vi "minimumSearch.vi"(7 "reset":bool, 11 "input":i16) -> (3 "minimum":i16)   [LabVIEW 2016]
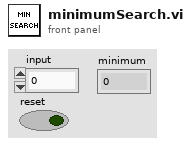
[diagram p1: front panel]
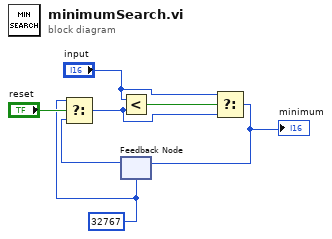
[diagram p0: block diagram]
diagram:
  w1 = i16 32767
  n1 = feedback #1(w1) -> (w5:i16)
  n2 = Select(t=w1, s="reset", f=w5) -> (s? t:f=w3:i16)
  n3 = Less?(x="input", y=w3) -> (x < y?=w7:bool)
  n4 = Select(t="input", s=w7, f=w3) -> (s? t:f=w4:i16)
  "minimum" <- w4
  n5 = feedback-in #1(w4) -> ()
